vi "VariablesLocales_sinGlobales.vi"() -> ()   [LabVIEW 2020]
panel:
  out "Waveform Chart 2":dbl(graph)
  out "Waveform Chart":dbl(graph)
  in  "Boton de paro de ambas":bool
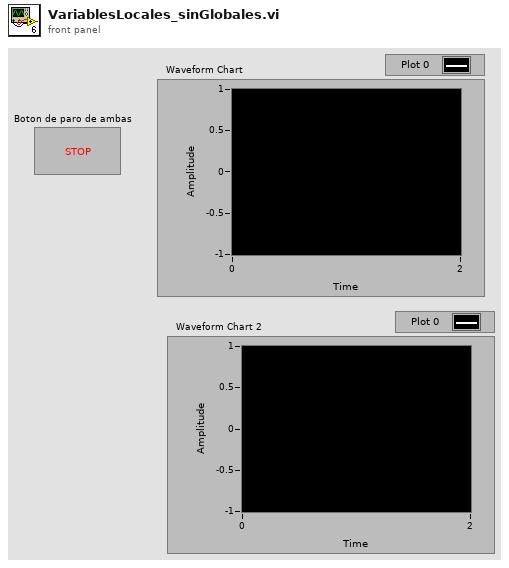
[diagram p1: front panel]
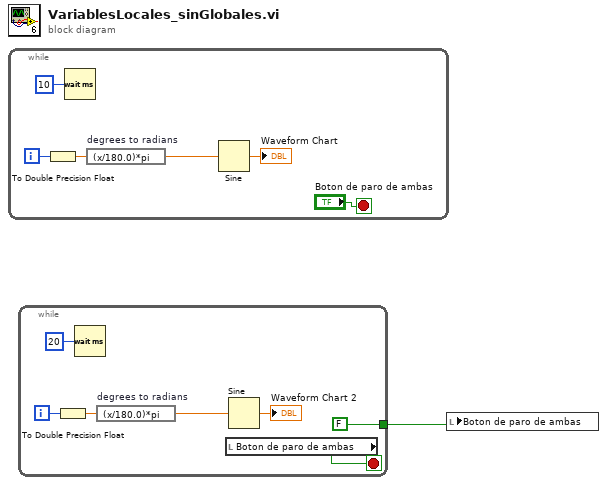
[diagram p0: block diagram]
diagram:
  n1 = while {
    i -> [w5]
    stop <- "Boton de paro de ambas" stop-if-true
    n2 = To Double Precision Float(number=w5) -> (double precision float=w4:dbl)
    n3 = Wait (ms)(milliseconds to wait=u32 10) -> ()  [unwired: 1 out]
    n4 = expression code="(x/180.0)*pi" "degrees to radians"(w4) -> (w6:dbl)
    n5 = Sine(x=w6) -> (sin(x)=→"Waveform Chart":dbl)
  }
  n6 = while {
    tunnel: [FALSE] -> w1
    i -> [w12]
    stop <- w9 stop-if-true
    n7 = To Double Precision Float(number=w12) -> (double precision float=w11:dbl)
    n8 = Wait (ms)(milliseconds to wait=u32 20) -> ()  [unwired: 1 out]
    n9 = expression code="(x/180.0)*pi" "degrees to radians"(w11) -> (w13:dbl)
    n10 = local read "Boton de paro de ambas"() -> (w9:bool)
    n11 = Sine(x=w13) -> (sin(x)=→"Waveform Chart 2":dbl)
  }
  n12 = local write "Boton de paro de ambas"(w1) -> ()
